vi "Camera.v2.vi"() -> ()   [LabVIEW 2015]
uses:
  CameraState.ctl
  Camera Properties.ctl
  <vilib>/vision/NI_Vision_Development_Module.lvlib
  CameraControlTypeDef.ctl
  Stack Track.ctl
  Stack_State.ctl
  ModeEnum.ctl
  <vilib>/DAQmx/create/channels.llb/DAQmx Create Channel (AO-Voltage-Basic).vi
  <vilib>/DAQmx/configure/timing.llb/DAQmx Timing (Sample Clock).vi
  WaveformModes.ctl
  <vilib>/DAQmx/write.llb/DAQmx Write (Digital 1D Wfm NChan NSamp).vi
  <vilib>/DAQmx/write.llb/DAQmx Write (Analog 1D Wfm NChan NSamp).vi
  Microscope Settings.ctl
panel:
  in  "Tab Control":enum32{"Camera Settings", "Recording"}(tab)
  in  "Scan":bool
  in  "Scan Continuously":bool
  in  "Camera Mode":T1(ring)
  in  "Slit Width /percent":dbl=100.0
  out "error IO":errorcluster
  in  "V Height":dbl=2048.0 min=4.0 max=2048.0 step=4.0
  in  "V Offset":dbl min=0.0 max=0.0 step=4.0
  in  "H Offset":dbl min=0.0 max=0.0 step=4.0
  in  "H Width":dbl min=4.0 max=2048.0 step=4.0
  in  "Exposure /ms":dbl=40.0 min=0.0010036691729323308 max=10.000004210526315 step=1e-08
  in  "Trigger Source":dbl(ring)=2.0 items=["Internal"=1.0, "External"=2.0]
  in  "Readout Direction":dbl(ring)=2.0 items=["Forward"=1.0, "Backward"=2.0]
  in  "Scanning Mode":dbl(ring)=12.0 items=["Full Frame"=1.0, "Slit Scanning"=12.0]
  in  "Advanced DCAM Controls":i32(listbox) caption="Multicolumn Listbox"
  in  "Mode":T2
  in  "FOV /um":dbl(slide) scale=-10.0..10.0
  in  "Mode":T3
  in  "Properties":T4=4211904 items=["SENSOR MODE"=4212128, "CCD MODE"=4212384, "READOUT MODE"=4211872, "ACTIVE VIEW INDEX"=4343136, "BITS PER CHANNEL"=4342976, "IMAGE PIXEL TYPE"=4343296, "BINNING"=4215968, "EXPOSURE TIME"=2049184, "CONTRAST GAIN"=3163312, "CONTRAST OFFSET"=3163328, "LIGHT MODE"=2114720, "SENSITIVITY"=2114992, "PHOTON IMAGING MODE"=2115200, "HIGH DYNAMIC RANGE MODE"=3163360, "WHITE BALANCE"=3163568, "TEMPERATURE"=2115232, "TEMPERATURE TARGET"=2115264, "SENSOR COOLER FAN"=2115296, "LINEBUNDLE HEIGHT"=4212192, "MECHANICAL SHUTTER"=2115488, "BACK FOCUS POSITION"=8422304, "TRIGGER CONNECTOR"=1066432, "TRIGGER SOURCE"=1066144, "OUTPUT TRIGGER SOURCE"=1852576, "TRIGGER GLOBAL EXPOSURE"=2049680, "FIRST TRIGGER BEHAVIOR"=2049696, "CHANNEL SYNC"=1852352, "READOUT DIRECTION"=4211904, "PRE HSYNC COUNT"=1852704, "INTERNAL LINE SPEED"=4191408, "INTERNAL LINE INVERVAL"=4191424]
  out "Image":T5(plugin-control)
  out "Histogram":T6(graph)
  in  "stop":bool
  in  "Calibration":bool
  in  "MultiD Scan":bool
  in  "Stage Controller":bool
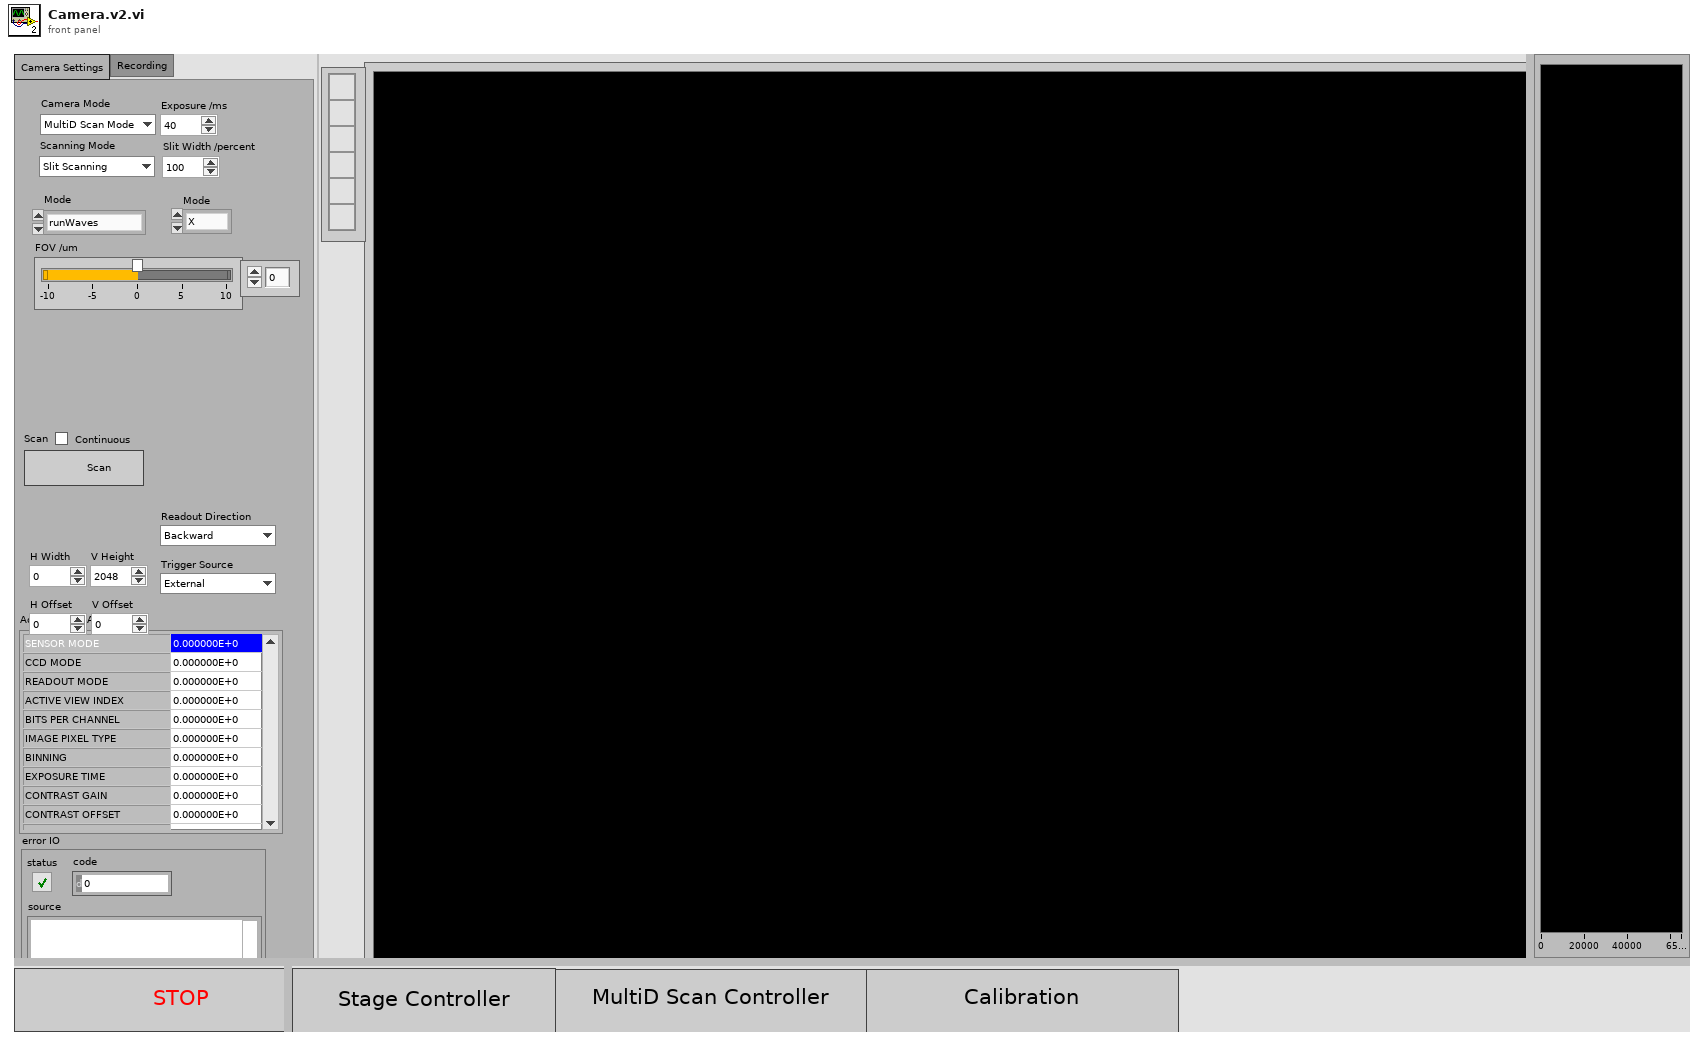
[diagram p1: front panel]
types:
  T1 = enum16{"MultiD Scan Mode", "2D Scan Mode", "Calibration Mode"}
  T2 = typedef "ModeEnum.ctl" = enum16{"runWaves", "generateWaves", "Idle", "stop"}
  T3 = typedef "WaveformModes.ctl" = enum16{"X", "XY", "XYZ", "XYZT", "XYZC"}
  T4 = typedef "Camera Properties.ctl" = u32
  T5 = typedef "IMAQ Image.ctl" = refnum<image>
  T6 = cluster{"Starting Value":sgl, "Incremental Value":sgl, "Histogram":u32[]}
  T7 = typedef "Microscope Settings.ctl" = cluster{"Mode":enum16{"X", "XY", "XYZ", "XYZT", "XYZC"}, "Piezo Position /um":dbl, "Exposure/ms":dbl, "Samples/millisecond":dbl, "Relax/ms":dbl}
  T8 = typedef "CameraControlTypeDef.ctl" = enum16{"IntervalLineInt", "Ram Record", "HardDisk Record", "Disengage Update", "Update", "Idle", "ROI", "Binning", "Scan Mode", "Trigger Mode", "Readout Mode", "Readout Direction", "Preview", "ROIWindow", "Trigger Source"}
  T9 = cluster{"height":u32, "width":u32, "datatype":u32}
  T10 = typedef "Stack_State.ctl" = cluster{"State":T11, "Stack Number":i32, "Image":u16[][], "Stacks":i32}
  T11 = typedef "Stack Track.ctl" = enum16{"Idle", "Display", "Start Sequence", "Read Disk", "STOP", "Collecting", "End"}
  T12 = typedef "CameraState.ctl" = enum16{"init", "active", "deinit"}
  T13 = typedef "Image Type" = u32
  T14 = cluster{"Value":i32, "Minimum":i32, "Maximum":i32, "Increment":i32}
  T15 = cluster{"Minimum":i32, "Maximum":i32, "Increment":i32}
  T16 = cluster{"Enum":T8, dbl, "timeout in ms (-1)":u32}
  T17 = cluster{"State":T11, "Timeout":i32, "Data 16":u16[][], "Timeout":i32}
  T18 = cluster{"Enum":T8, "Trigger Source":dbl, "timeout in ms (-1)":i32}
  T19 = cluster{"Enum":T8, "Exposure /ms":dbl, "Parameter":u32}
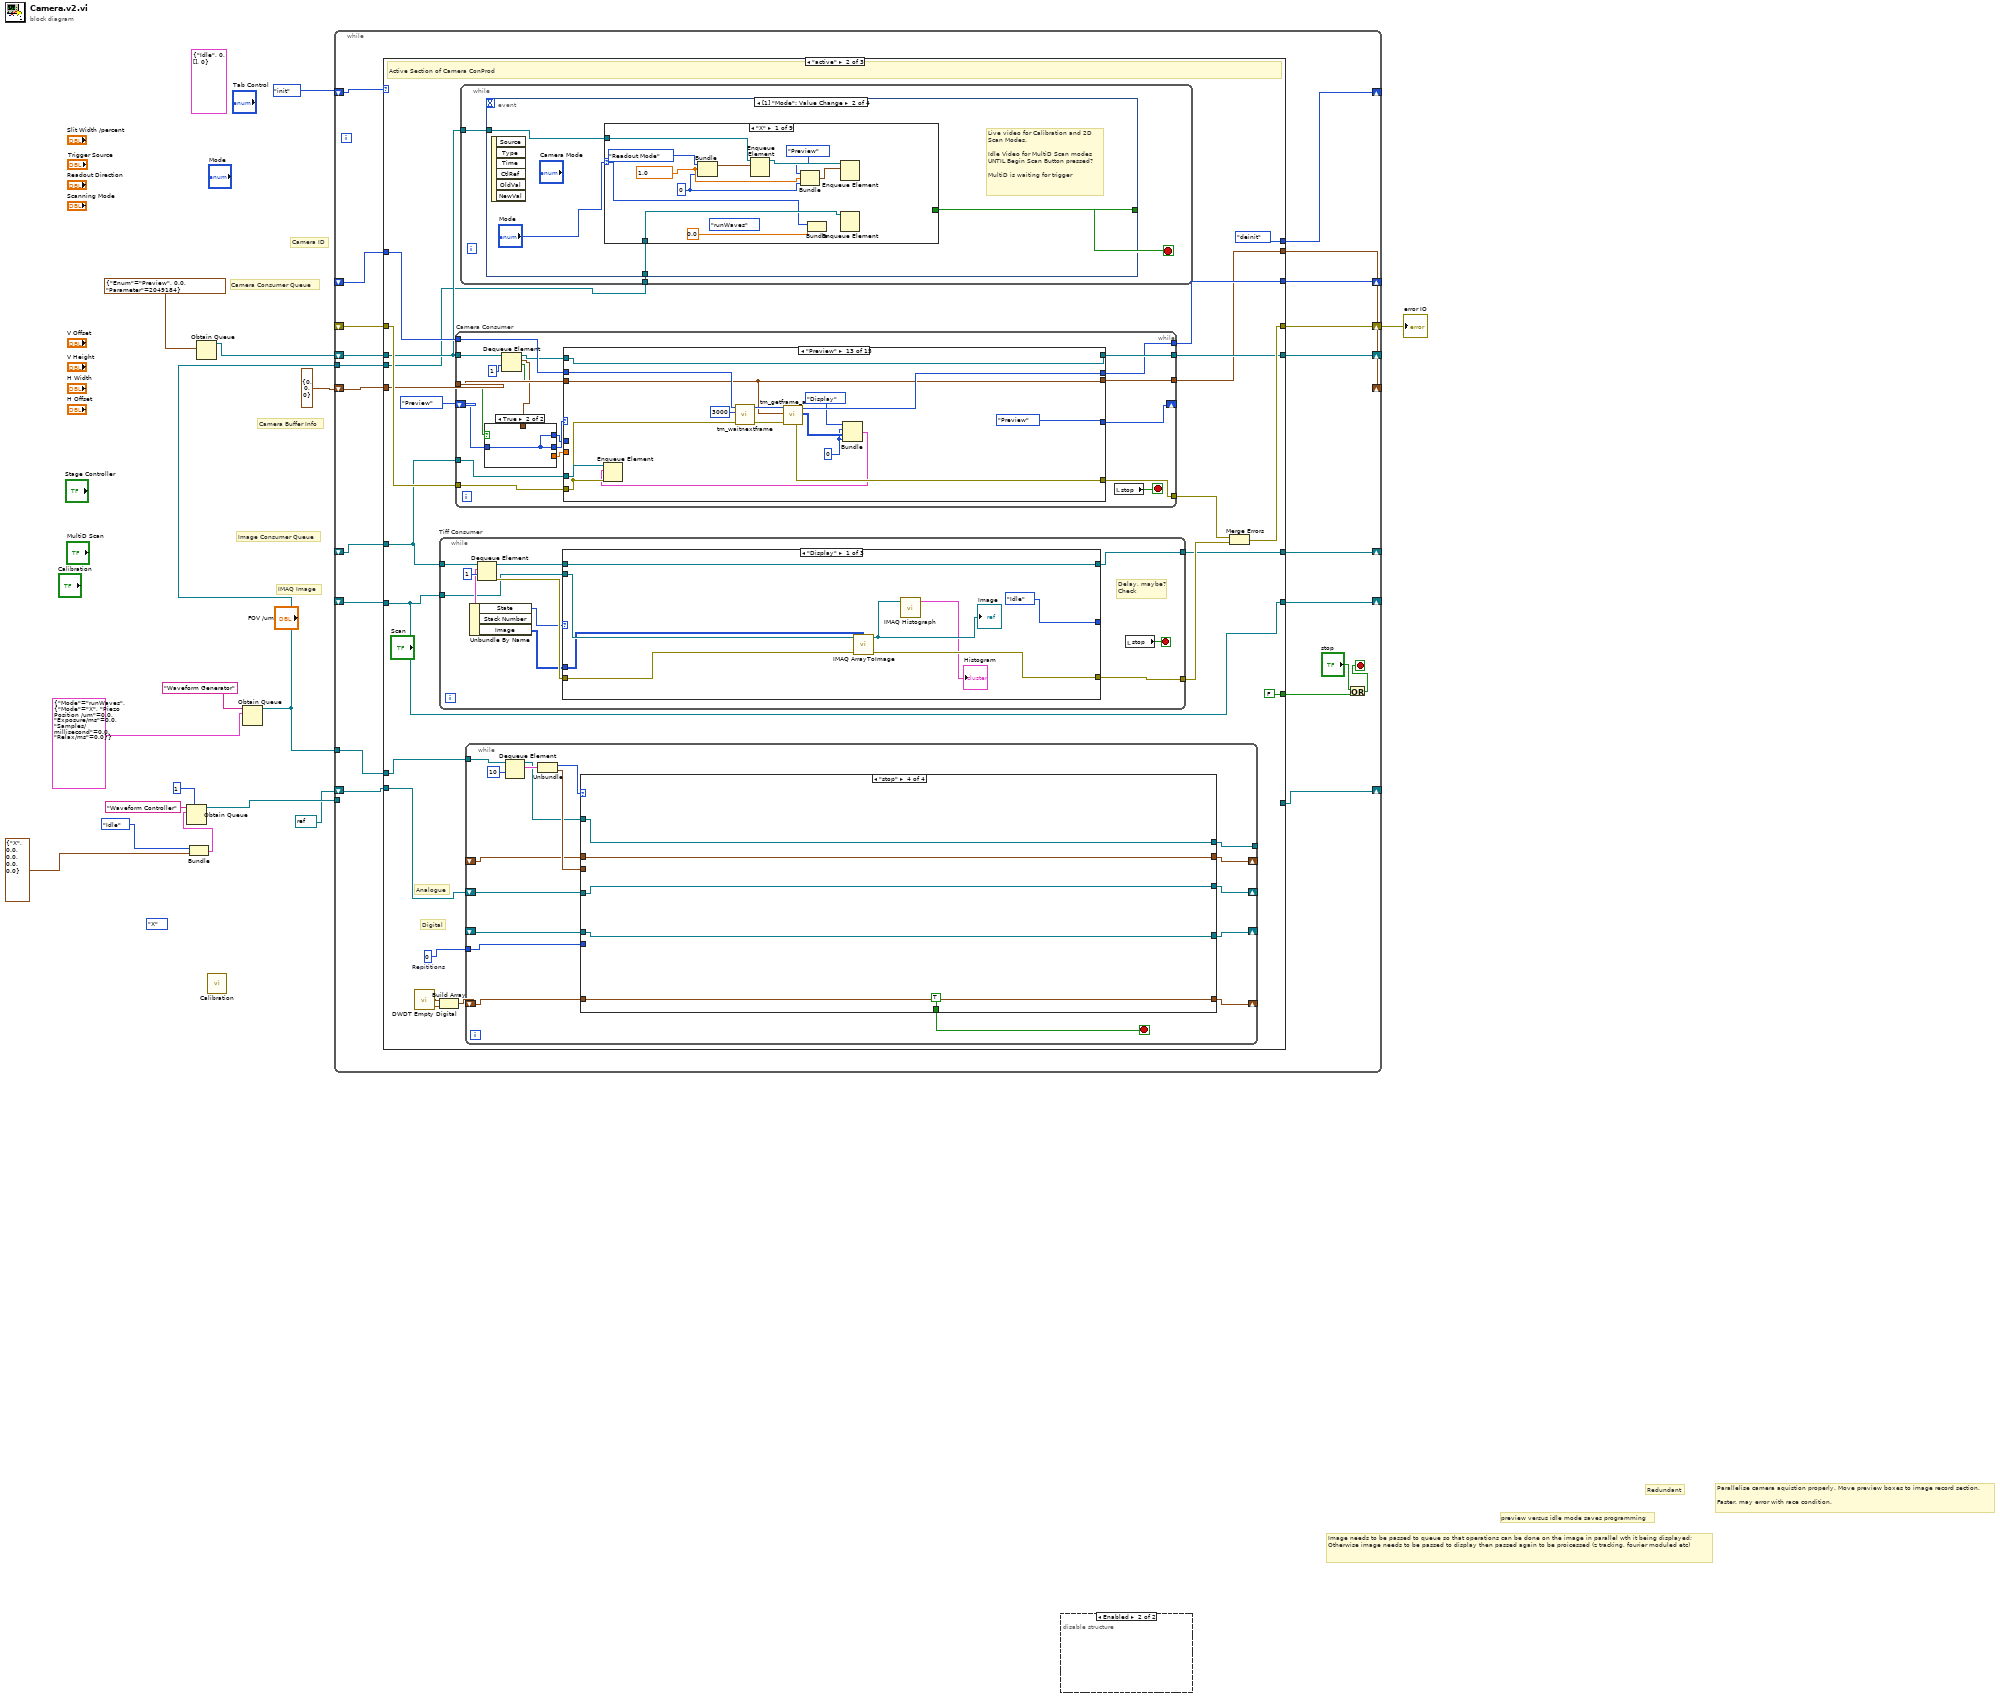
[diagram p0: block diagram]
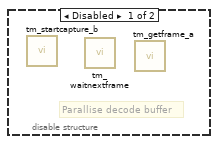
[diagram p2: hidden frame]
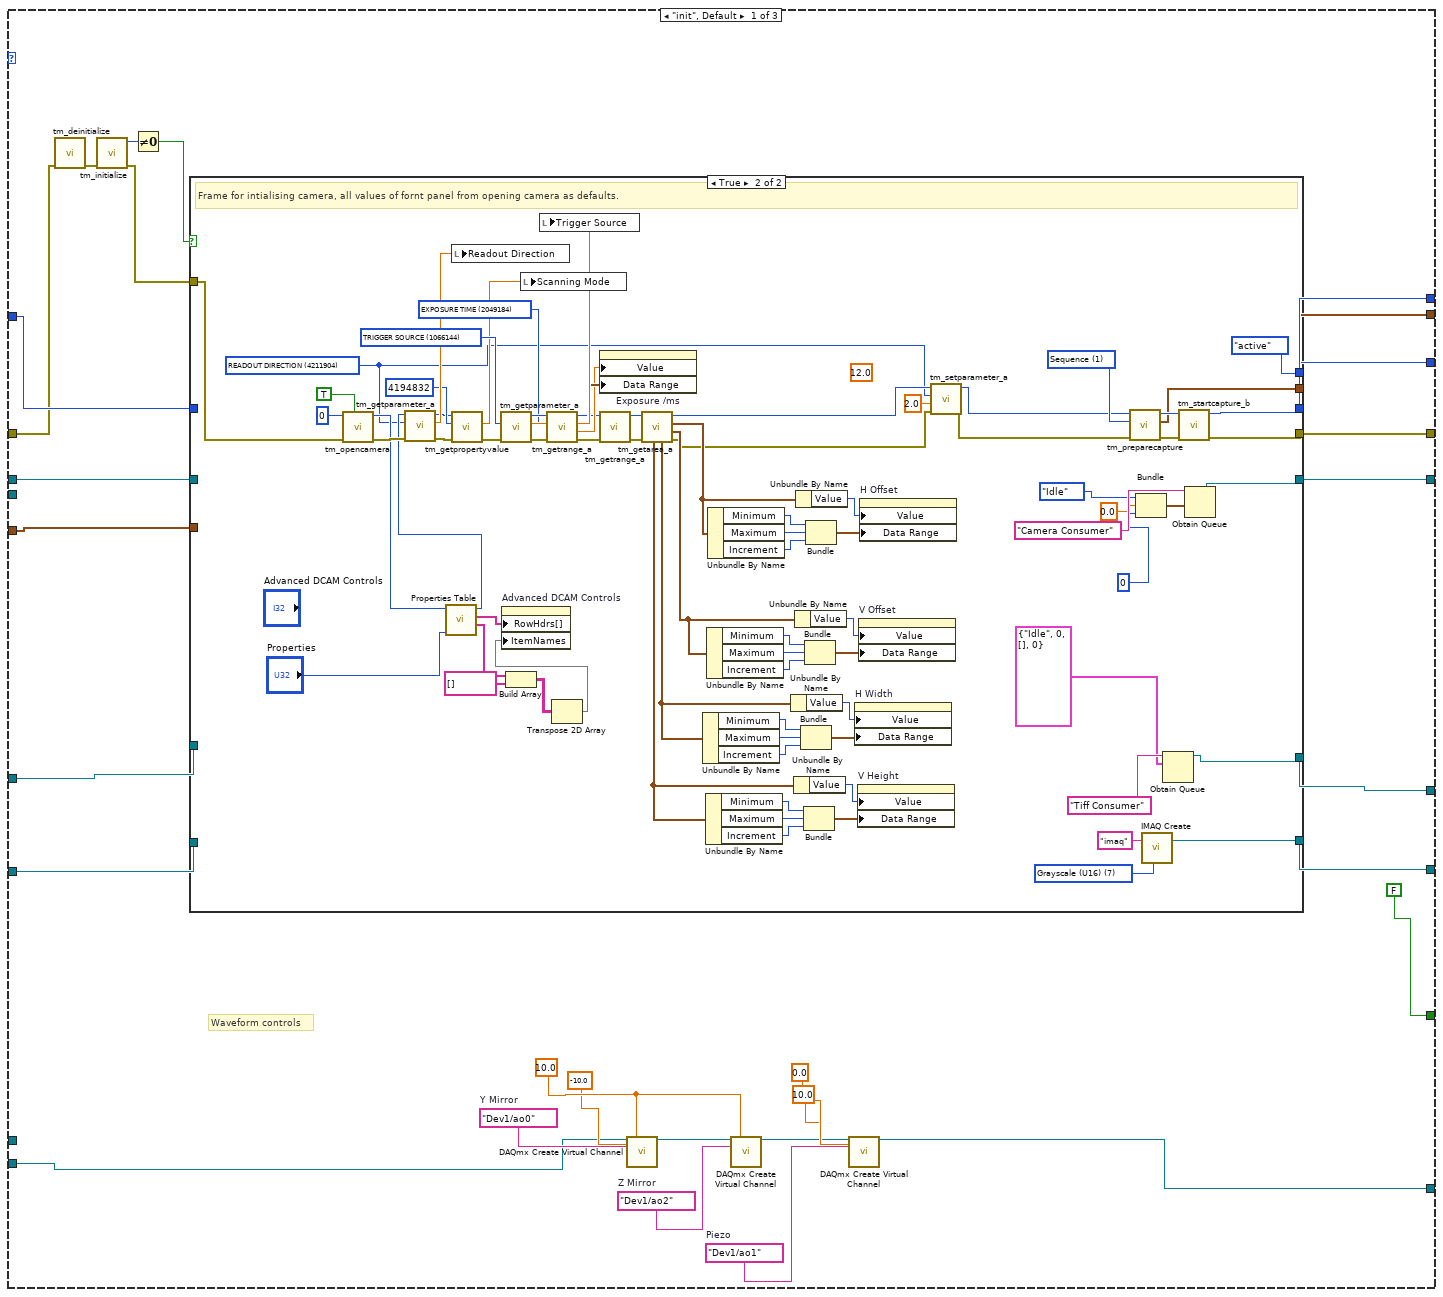
[diagram p3: hidden frame]
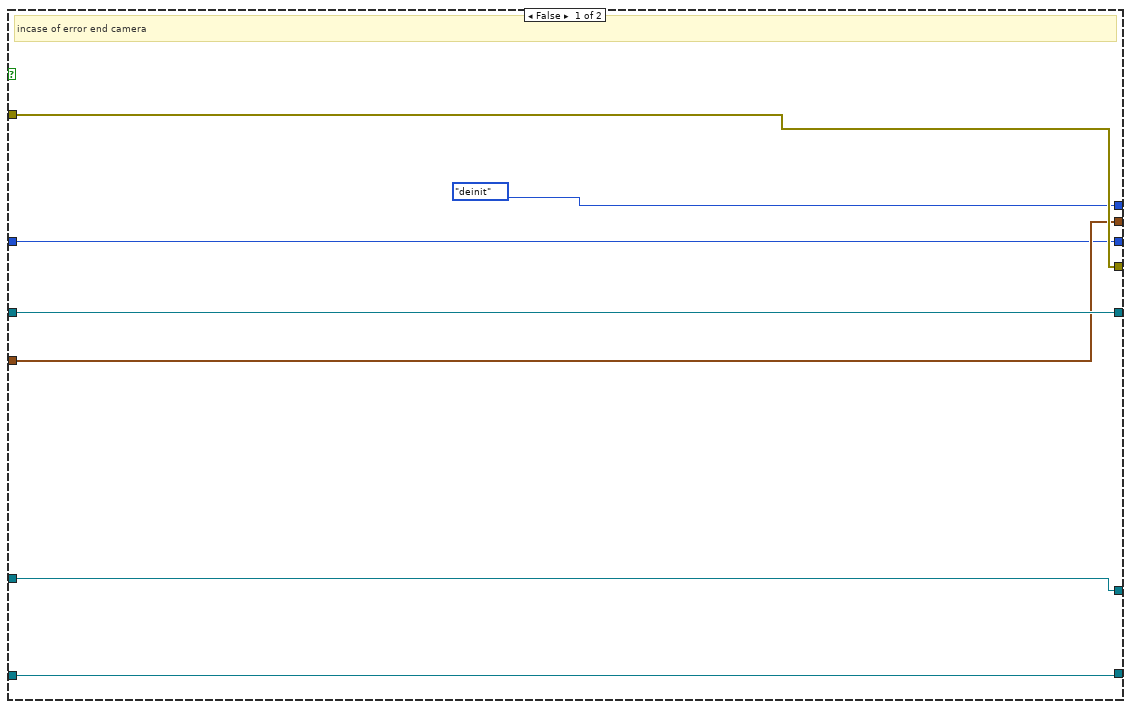
[diagram p4: hidden frame]
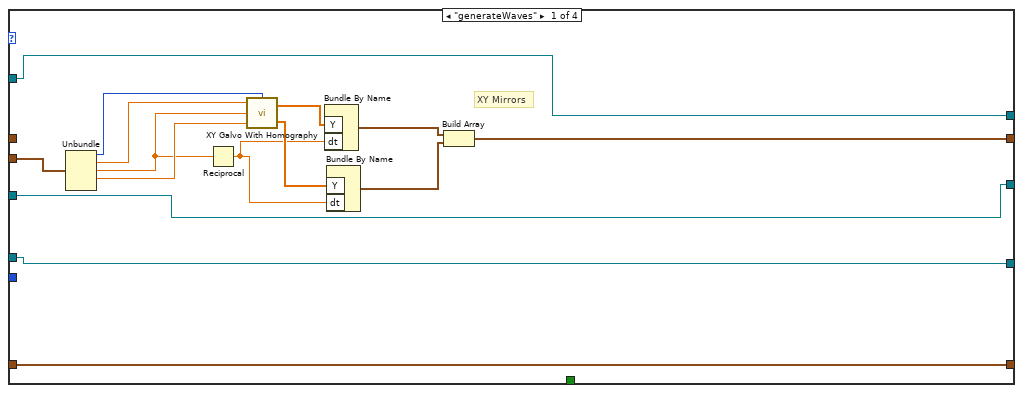
[diagram p5: hidden frame]
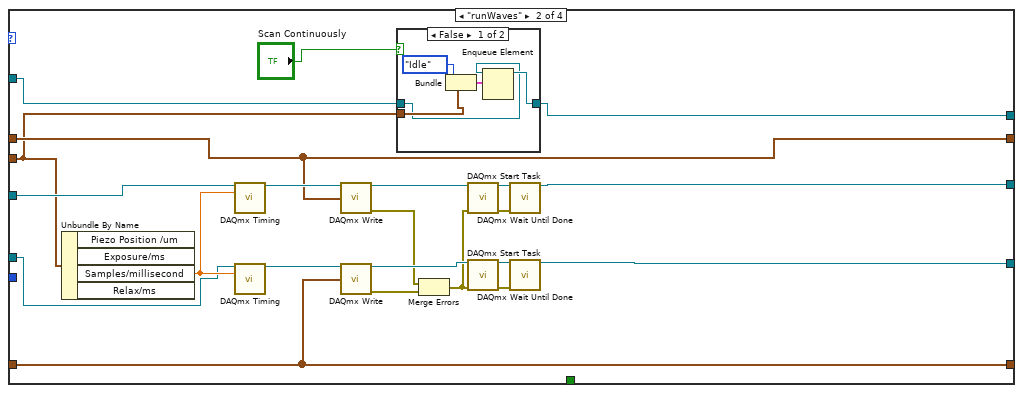
[diagram p6: hidden frame]
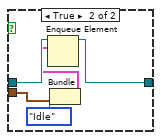
[diagram p7: hidden frame]
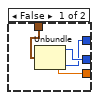
[diagram p11: hidden frame]
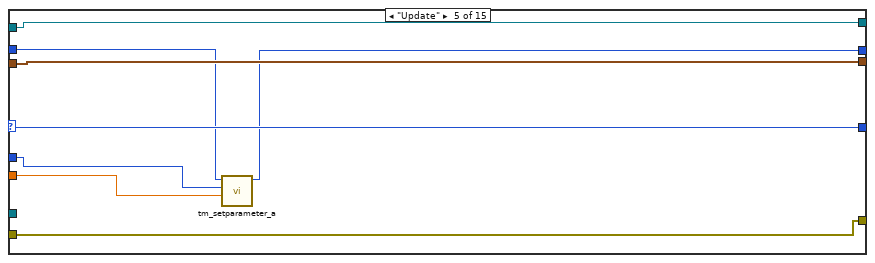
[diagram p16: hidden frame]
diagram:
  (unwired) WaveformModes."X"
  (unwired) T10 {"State"=enum."Idle", "Stack Number"=0, "Image"=[], "Stacks"=0} ("input cluster")
  # "IMAQ Image"
  # "Camera Buffer Info"
  # "Image needs to be passed to queue so that operations can be done on the image in parallel wth it being displayed;\nOtherwise image needs to be passed to display then passed again to be proicessed (z tracking, fourier moduled etc)"
  # "preview versus idle mode saves programming"
  # "Parallelise camera aquistion properly. Move preview boxes to image record section.\n\nFaster. may error with race condition."
  # "Redundant"
  # "Image Consumer Queue"
  # "Camera Consumer Queue"
  # "Camera ID"
  n1 = Bundle("Mode"=ModeEnum."Idle", T7 {"Mode"=enum."X", "Piezo Position /um"=0.0, "Exposure/ms"=0.0, "Samples/millisecond"=0.0, "Relax/ms"=0.0}) -> (w6:cluster{"Mode":T2, T7})  [unwired: 1 in]
  n2 = Obtain Queue(max queue size (-1, unlimited)=1, name (unnamed)="Waveform Controller", element data type=w6) -> (queue out=w3:refnum<queue>)  [unwired: 2 in, 2 out]
  n3 = Obtain Queue(element data type=cluster{"Enum":T8, dbl, "Parameter":u32} {"Enum"=enum."Preview", 0.0, "Parameter"=2049184}) -> (queue out=w10:refnum<queue>)  [unwired: 4 in, 2 out]
  n4 = call "Calibration.vi"() -> ()  [unwired: 1 in, 1 out]
  n5 = Obtain Queue(name (unnamed)="Waveform Generator", element data type=cluster{"Mode":T2, T7} {"Mode"=enum."runWaves", {"Mode"=enum."X", "Piezo Position /um"=0.0, "Exposure/ms"=0.0, "Samples/millisecond"=0.0, "Relax/ms"=0.0}}) -> (queue out=w9:refnum<queue>)  [unwired: 3 in, 2 out]
  n6 = while {
    shift-right: [w36] -> _
    shift-left: CameraState."init" -> [w35]
    shift-right: [w34] -> _
    shift-left: _ -> [w33]
    shift-right: [w32] -> w14
    shift-left: _ -> [w31]
    shift-right: [w29] -> _
    shift-left: _ -> [w28]
    shift-right: [w30] -> _
    shift-left: w10 -> [w27]
    shift-right: [w23] -> _
    shift-left: T9 {"height"=0, "width"=0, "datatype"=0} ("Buffer Info") -> [w22]
    shift-right: [w21] -> _
    shift-left: _ -> [w20]
    tunnel: w9 -> [w19]
    tunnel: w9 -> [w18]
    tunnel: w3 -> [_]
    shift-right: [w17] -> _
    shift-left: refnum<k21> refnum ("Mirror Z 2") -> [w16]
    stop <- w25 stop-if-true
    n7 = case shown="\"active\"" w35 {
      tunnel: [w61 CameraState."deinit" CameraState."init"] -> w36
      tunnel: [w60 w171 w445] -> w34
      tunnel: w33 -> [w38 w172 w445]
      tunnel: [w59 w170 w448] -> w32
      tunnel: w31 -> [w37 w164 w449]
      tunnel: [w58 w167 w442] -> w30
      tunnel: [w57 w166 w443] -> w29
      tunnel: w28 -> [w55 w159 w443]
      tunnel: w27 -> [w56 w157 w442]
      tunnel: [FALSE ("stop") FALSE ("stop") TRUE ("stop")] -> w24
      tunnel: [w53 w162 w440] -> w23
      tunnel: w22 -> [w52 w161 w440]
      tunnel: w20 -> [w50 w158 w439]
      tunnel: [w51 w158 w439] -> w21
      tunnel: w19 -> [_ w151 _]
      tunnel: w18 -> [_ w156 _]
      tunnel: [w42 _ w437] -> w17
      tunnel: w16 -> [w39 w152 w437]
      frame "init", Default {
        w45 = tag "Dev1/ao1"  # Piezo
        w46 = tag "Dev1/ao2"  # Z Mirror
        w47 = tag "Dev1/ao0"  # Y Mirror
        w49 = 10.0 ("maximum value")
        # "Waveform controls"
        n8 = call "tm_deinitialize.vi"("error in (no error)"=w37) -> ("error out"=w65:errorcluster)  [unwired: 10 in]
        n9 = call "tm_initialize.vi"("error in (no error)"=w65) -> ("error out"=w62:errorcluster, "Number Of Cameras"=w64:u32)  [unwired: 7 in, 2 out]
        n10 = Not Equal To 0?(x=w64) -> (x != 0?=w63:bool)
        n11 = case shown="True" w63 {
          tunnel: w62 -> [w72 w144]
          tunnel: [CameraState."deinit" CameraState."active"] -> w61
          tunnel: [w72 w127] -> w59
          tunnel: [w67 w125] -> w60
          tunnel: [w70 w99] -> w58
          tunnel: [w69 w97] -> w57
          tunnel: w56 -> [w70 _]
          tunnel: w55 -> [w69 _]
          tunnel: [w68 w87] -> w53
          tunnel: w52 -> [w68 _]
          tunnel: w38 -> [w67 _]
          tunnel: [w66 w84] -> w51
          tunnel: w50 -> [w66 _]
          frame False {
            # "incase of error end camera"
          }
          frame True {
            (unwired) 12.0 ("Value in")
            w86 = T13 7 items=["Grayscale (U8)", "Grayscale (I16)", "Grayscale (SGL)", "Complex (CSG)", "RGB (U32)", "HSL (U32)", "RGB (U64)", "Grayscale (U16)"] ("Image Type")
            w129 = 1 items=["Snap", "Sequence"] ("Capture mode")
            w141 = u32 2049184 items=["SENSOR MODE"=4212128, "CCD MODE"=4212384, "READOUT MODE"=4211872, "ACTIVE VIEW INDEX"=4343136, "BITS PER CHANNEL"=4342976, "IMAGE PIXEL TYPE"=4343296, "BINNING"=4215968, "EXPOSURE TIME"=2049184, "CONTRAST GAIN"=3163312, "CONTRAST OFFSET"=3163328, "LIGHT MODE"=2114720, "SENSITIVITY"=2114992, "PHOTON IMAGING MODE"=2115200, "HIGH DYNAMIC RANGE MODE"=3163360, "WHITE BALANCE"=3163568, "TEMPERATURE"=2115232, "TEMPERATURE TARGET"=2115264, "SENSOR COOLER FAN"=2115296, "LINEBUNDLE HEIGHT"=4212192, "MECHANICAL SHUTTER"=2115488, "BACK FOCUS POSITION"=8422304, "TRIGGER CONNECTOR"=1066432, "TRIGGER SOURCE"=1066144, "OUTPUT TRIGGER SOURCE"=1852576, "TRIGGER GLOBAL EXPOSURE"=2049680, "FIRST TRIGGER BEHAVIOR"=2049696, "CHANNEL SYNC"=1852352, "READOUT DIRECTION"=4211904, "PRE HSYNC COUNT"=1852704, "INTERNAL LINE SPEED"=4191408, "INTERNAL LINE INVERVAL"=4191424] ("Parameter")
            w79 = T4 4211904 items=["SENSOR MODE"=4212128, "CCD MODE"=4212384, "READOUT MODE"=4211872, "ACTIVE VIEW INDEX"=4343136, "BITS PER CHANNEL"=4342976, "IMAGE PIXEL TYPE"=4343296, "BINNING"=4215968, "EXPOSURE TIME"=2049184, "CONTRAST GAIN"=3163312, "CONTRAST OFFSET"=3163328, "LIGHT MODE"=2114720, "SENSITIVITY"=2114992, "PHOTON IMAGING MODE"=2115200, "HIGH DYNAMIC RANGE MODE"=3163360, "WHITE BALANCE"=3163568, "TEMPERATURE"=2115232, "TEMPERATURE TARGET"=2115264, "SENSOR COOLER FAN"=2115296, "LINEBUNDLE HEIGHT"=4212192, "MECHANICAL SHUTTER"=2115488, "BACK FOCUS POSITION"=8422304, "TRIGGER CONNECTOR"=1066432, "TRIGGER SOURCE"=1066144, "OUTPUT TRIGGER SOURCE"=1852576, "TRIGGER GLOBAL EXPOSURE"=2049680, "FIRST TRIGGER BEHAVIOR"=2049696, "CHANNEL SYNC"=1852352, "READOUT DIRECTION"=4211904, "PRE HSYNC COUNT"=1852704, "INTERNAL LINE SPEED"=4191408, "INTERNAL LINE INVERVAL"=4191424] ("Parameter")
            w147 = u32 1066144 items=["SENSOR MODE"=4212128, "CCD MODE"=4212384, "READOUT MODE"=4211872, "ACTIVE VIEW INDEX"=4343136, "BITS PER CHANNEL"=4342976, "IMAGE PIXEL TYPE"=4343296, "BINNING"=4215968, "EXPOSURE TIME"=2049184, "CONTRAST GAIN"=3163312, "CONTRAST OFFSET"=3163328, "LIGHT MODE"=2114720, "SENSITIVITY"=2114992, "PHOTON IMAGING MODE"=2115200, "HIGH DYNAMIC RANGE MODE"=3163360, "WHITE BALANCE"=3163568, "TEMPERATURE"=2115232, "TEMPERATURE TARGET"=2115264, "SENSOR COOLER FAN"=2115296, "LINEBUNDLE HEIGHT"=4212192, "MECHANICAL SHUTTER"=2115488, "BACK FOCUS POSITION"=8422304, "TRIGGER CONNECTOR"=1066432, "TRIGGER SOURCE"=1066144, "OUTPUT TRIGGER SOURCE"=1852576, "TRIGGER GLOBAL EXPOSURE"=2049680, "FIRST TRIGGER BEHAVIOR"=2049696, "CHANNEL SYNC"=1852352, "READOUT DIRECTION"=4211904, "PRE HSYNC COUNT"=1852704, "INTERNAL LINE SPEED"=4191408, "INTERNAL LINE INVERVAL"=4191424] ("Parameter")
            # "Frame for intialising camera, all values of fornt panel from opening camera as defaults."
            n12 = call "tm_opencamera.vi"("Force Open"=TRUE, "error in (no error)"=w144, "Camera Index"=u32 0) -> ("error out"=w148:errorcluster, "Handle out"=w95:u32)  [unwired: 6 in, 1 out]
            n13 = call "Properties Table.vi"("Properties"="Properties", "Handle In"=w95) -> ("Value Stirngs Out"=w92:string[], "Row Headers"=w93:string[], "Handle Out"=w94:u32)  [unwired: 3 in, 1 out]
            n14 = call "tm_getparameter_a.vi"("error in (no error)"=w148, "Parameter"=w79, "Handle in"=w94) -> ("error out"=w130:errorcluster, "Value out"=w145:dbl, "Handle out"=w133:u32)  [unwired: 6 in]
            n15 = local write "Readout Direction"(w145) -> ()
            n16 = call "tm_getpropertyvalue.vi"("error in (no error)"=w130, "Property ID"=u32 4194832, "Handle in"=w133) -> ("error out"=w131:errorcluster, "Value in"=w132:sgl)  [unwired: 6 in, 1 out]
            n17 = call "tm_getparameter_a.vi"("error in (no error)"=w131, "Parameter"=w147) -> ("error out"=w142:errorcluster, "Value out"=w146:dbl, "Handle out"=w143:u32)  [unwired: 7 in]
            n18 = Build Array(w92, string[] [] ("element")) -> (w90:string[][])
            n19 = local write "Scanning Mode"(w132) -> ()
            n20 = local write "Trigger Source"(w146) -> ()
            n21 = call "tm_getrange_a.vi"("error in (no error)"=w142, "Parameter"=w141, "Handle in"=w143) -> ("error out"=w137:errorcluster, "default"=w139:dbl, "Range"=w140:cluster{"min":dbl, "max":dbl, "step":dbl}, "Handle out"=w138:u32)  [unwired: 2 in, 3 out]
            n22 = Transpose 2D Array(2D array=w90) -> (transposed array=w89:string[][])
            n23 = property on="Advanced DCAM Controls" class="MCListbox (strict)"("RowHdrs[]"=w93, "ItemNames"=w89) -> ()  [unwired: 2 in, 2 out]
            n24 = property on="Exposure /ms" class="DigNum (strict)"("Value"=w139, "Data Range"=w140) -> ()  [unwired: 2 in, 2 out]
            n25 = call "tm_getrange_a.vi"("error in (no error)"=w137, "Handle in"=w138) -> ("error out"=w136:errorcluster, "Handle out"=w135:u32)  [unwired: 3 in, 5 out]
            n26 = call "tm_getarea_a.vi"("error in (no error)"=w136, "Handle in"=w135) -> ("error out"=w81:errorcluster, "V Offset"=w101:T14, "H Offset"=w124:T14, "Handle out"=w83:u32, "H Width"=w102:T14, "V Width"=w103:T14)  [unwired: 4 in]
            n27 = Unbundle By Name(w102) -> ("Minimum"=w113:i32, "Maximum"=w112:i32, "Increment"=w111:i32)
            n28 = Unbundle By Name(w103) -> ("Minimum"=w104:i32, "Maximum"=w105:i32, "Increment"=w106:i32)
            n29 = Unbundle By Name(w101) -> ("Minimum"=w114:i32, "Maximum"=w115:i32, "Increment"=w116:i32)
            n30 = Unbundle By Name(w124) -> ("Minimum"=w123:i32, "Maximum"=w122:i32, "Increment"=w121:i32)
            n31 = Unbundle By Name(w102) -> ("Value"=w109:i32)
            n32 = Unbundle By Name(w103) -> ("Value"=w108:i32)
            n33 = Unbundle By Name(w101) -> ("Value"=w118:i32)
            n34 = Unbundle By Name(w124) -> ("Value"=w119:i32)
            n35 = Bundle("Minimum"=w113, "Maximum"=w112, "Increment"=w111) -> (w110:T15)  [unwired: 1 in]
            n36 = Bundle("Minimum"=w104, "Maximum"=w105, "Increment"=w106) -> (w107:T15)  [unwired: 1 in]
            n37 = Bundle("Minimum"=w114, "Maximum"=w115, "Increment"=w116) -> (w117:T15)  [unwired: 1 in]
            n38 = Bundle("Minimum"=w123, "Maximum"=w122, "Increment"=w121) -> (w120:T15)  [unwired: 1 in]
            n39 = property on="H Width" class="DigNum (strict)"("Value"=w109, "Data Range"=w110) -> ()  [unwired: 2 in, 2 out]
            n40 = property on="V Height" class="DigNum (strict)"("Value"=w108, "Data Range"=w107) -> ()  [unwired: 2 in, 2 out]
            n41 = property on="V Offset" class="DigNum (strict)"("Value"=w118, "Data Range"=w117) -> ()  [unwired: 2 in, 2 out]
            n42 = property on="H Offset" class="DigNum (strict)"("Value"=w119, "Data Range"=w120) -> ()  [unwired: 2 in, 2 out]
            n43 = call "tm_setparameter_a.vi"("error in (no error)"=w81, "Value in"=2.0, "Parameter"=w79, "Handle in"=w83) -> ("error out"=w80:errorcluster, "Handle out"=w82:u32)  [unwired: 6 in]
            n44 = call "tm_preparecapture.vi"("error in (no error)"=w80, "Capture mode"=w129, "Handle in"=w82) -> ("error out"=w128:errorcluster, "Buffer Info"=w87:T9, "Handle out"=w126:u32)  [unwired: 5 in, 1 out]
            n45 = Bundle("Enum"=CameraControlTypeDef."Idle", 0.0, "timeout in ms (-1)"=u32 0) -> (w75:T16)  [unwired: 1 in]
            n46 = call "IMAQ Create"("Image Name"="imaq", "Image Type"=w86) -> ("New Image"=w84:T5)  [unwired: 3 in, 1 out]
            n47 = Obtain Queue(name (unnamed)="Tiff Consumer", element data type=T10 {"State"=enum."Idle", "Stack Number"=0, "Image"=[], "Stacks"=0} ("input cluster")) -> (queue out=w97:refnum<queue>)  [unwired: 3 in, 2 out]
            n48 = call "tm_startcapture_b.vi"("error in (no error)"=w128, "Handle in"=w126) -> ("error out"=w127:errorcluster, "Handle out"=w125:u32)  [unwired: 8 in]
            n49 = Obtain Queue(name (unnamed)="Camera Consumer", element data type=w75) -> (queue out=w99:refnum<queue>)  [unwired: 3 in, 2 out]
          }
        }
        n50 = call-poly <vilib>:"DAQmx Create Virtual Channel.vi"("task in"=w39, "maximum value"=w49, "minimum value"=-10.0, "physical channels"=w47) -> ("task out"=w41:refnum<k21>)  [unwired: 10 in, 1 out]
        n51 = call-poly <vilib>:"DAQmx Create Virtual Channel.vi"("task in"=w41, "maximum value"=w49, "physical channels"=w46) -> ("task out"=w40:refnum<k21>)  [unwired: 11 in, 1 out]
        n52 = call-poly <vilib>:"DAQmx Create Virtual Channel.vi"("task in"=w40, "maximum value"=10.0 ("minimum value"), "minimum value"=0.0 ("maximum value"), "physical channels"=w45) -> ("task out"=w42:refnum<k21>)  [unwired: 10 in, 1 out]
      }
      frame "active" {
        w155 = 0  # Repititions
        # "Digital"
        # "Analogue"
        # "Active Section of Camera ConProd"
        n53 = call <vilib>:"DWDT Empty Digital.vi"() -> ("digital waveform out"=w153:digitalwaveform)  [unwired: 5 in]
        n54 = while "Tiff Consumer" {
          tunnel: [w251] -> w169
          tunnel: [w254] -> w166
          tunnel: w159 -> [w256]
          tunnel: w158 -> [w248]
          stop <- w258 stop-if-true
          # "Delay, maybe?\nCheck"
          n55 = Dequeue Element(queue=w256, timeout in ms (-1)=1) -> (queue out=w253:refnum<queue>, element=w255:T10, error out=w252:errorcluster)  [unwired: 1 in, 1 out]
          n56 = Unbundle By Name(w255) -> ("State"=w249:T11, "Image"=w250:u16[][])  [unwired: 1 out]
          n57 = case shown="\"Display\"" w249 {
            selector: w249 -> [_ w269 w270]
            tunnel: [w266 w268 w271] -> w254
            tunnel: w253 -> [w266 w268 w271]
            tunnel: [Stack_Track."Idle" ("State") w269 w270] -> _
            tunnel: w250 -> [w261 _ _]
            tunnel: w248 -> [w265 _ _]
            tunnel: w252 -> [w264 w267 w272]
            tunnel: [w263 w267 w272] -> w251
            frame "Display" {
              n58 = call "IMAQ ArrayToImage"("Image Pixels (U16)"=w261, "error in (no error)"=w264, "Image"=w265) -> ("error out"=w263:errorcluster, "Image Out"=w260:T5)  [unwired: 7 in]
              "Image" <- w260
              n59 = call "IMAQ Histograph"("Image"=w260) -> ("Histogram Graph"=→"Histogram":T6)  [unwired: 7 in, 3 out]
            }
            frame "Idle", Default {
            }
            frame "Start Sequence" {
            }
          }
          n60 = local read "stop"() -> (w258:bool)
        }
        n61 = Build Array(w153, w153) -> (w154:digitalwaveform[])
        n62 = while "Camera Consumer" {
          tunnel: w164 -> [w289]
          tunnel: w172 -> [w286]
          tunnel: [w285] -> w171
          tunnel: [w288] -> w168
          tunnel: w157 -> [w281]
          tunnel: [w290] -> w167
          shift-right: [w287] -> _
          shift-left: CameraControlTypeDef."Preview" ("Enum") -> [w277]
          tunnel: [w284] -> w162
          tunnel: w161 -> [w283]
          tunnel: w159 -> [w276]
          stop <- w291 stop-if-true
          n63 = Dequeue Element(queue=w281, timeout in ms (-1)=1) -> (queue out=w280:refnum<queue>, element=w275:cluster{"Enum":T8, dbl, "Parameter":u32}, timed out?=w279:bool)  [unwired: 1 in, 1 out]
          n64 = case shown="True" w279 {
            tunnel: [w294 w296] -> w278
            tunnel: w277 -> [_ w296]
            tunnel: w275 -> [w295 _]
            tunnel: [w293 _] -> w274
            tunnel: [w292 w296] -> w273
            frame False {
              n65 = Unbundle(w295) -> ("Enum"=w294:T8, w293:dbl, "Parameter"=w292:u32)
            }
            frame True {
            }
          }
          n66 = case shown="\"Preview\"" w278 {
            selector: w278 -> [w300 w305 w310 w315 w323 w328 w333 w338 w343 w348 w353 w358 _ w377 _]
            tunnel: w280 -> [w299 w306 w311 w316 w324 w329 w334 w339 w344 w349 w354 w359 w374 w379 w384]
            tunnel: [w299 w306 w311 w316 w324 w329 w334 w339 w344 w349 w354 w359 w374 w379 w384] -> w290
            tunnel: w289 -> [w301 w304 w309 w314 w322 w327 w332 w337 w342 w347 w352 w357 w364 w376 w382]
            tunnel: [w301 w304 w309 w314 w322 w327 w332 w337 w342 w347 w352 w357 w368 w376 w382] -> w288
            tunnel: [w300 w305 w310 w315 w323 w328 w333 w338 w343 w348 w353 w358 CameraControlTypeDef."Preview" ("Enum") w377 CameraControlTypeDef."Preview" ("Enum")] -> w287
            tunnel: w286 -> [w298 w303 w308 w313 w320 w326 w331 w336 w341 w346 w351 w356 w372 w378 w383]
            tunnel: [w298 w303 w308 w313 w319 w326 w331 w336 w341 w346 w351 w356 w370 w378 w383] -> w285
            tunnel: [w297 w302 w307 w312 w321 w325 w330 w335 w340 w345 w350 w355 w366 w375 w381] -> w284
            tunnel: w283 -> [w297 w302 w307 w312 w321 w325 w330 w335 w340 w345 w350 w355 w366 w375 w381]
            tunnel: w276 -> [_ _ _ _ _ _ _ _ _ _ _ _ w365 _ _]
            tunnel: w274 -> [_ _ _ _ w317 _ _ _ _ _ _ _ _ _ _]
            tunnel: w273 -> [_ _ _ _ w318 _ _ _ _ _ _ _ _ _ _]
            frame "IntervalLineInt" {
            }
            frame "Ram Record" {
            }
            frame "HardDisk Record" {
            }
            frame "Disengage Update" {
            }
            frame "Update" {
              n67 = call "tm_setparameter_a.vi"("Value in"=w317, "Parameter"=w318, "Handle in"=w320) -> ("Handle out"=w319:u32)  [unwired: 7 in, 1 out]
            }
            frame "Idle", Default {
            }
            frame "ROI" {
            }
            frame "Binning" {
            }
            frame "Scan Mode" {
            }
            frame "Trigger Mode" {
            }
            frame "Readout Mode" {
            }
            frame "Readout Direction" {
            }
            frame "Preview" {
              w361 = 0 ("Timeout")
              n68 = call "tm_waitnextframe.vi"("error in (no error)"=w364, "Timeout"=3000, "Handle in"=w372) -> ("error out"=w369:errorcluster, "Handle out"=w371:u32)  [unwired: 5 in, 2 out]
              n69 = call "tm_getframe_a.vi"("error in (no error)"=w369, "Buffer Info"=w366, "Handle in"=w371) -> ("error out"=w368:errorcluster, "Data 16"=w362:u16[][], "Handle out"=w370:u32)  [unwired: 4 in, 2 out]
              n70 = Bundle("State"=Stack_Track."Display", "Timeout"=w361, "Data 16"=w362, "Timeout"=w361) -> (w360:T17)  [unwired: 1 in]
              n71 = Enqueue Element(queue=w365, element=w360, error in (no error)=w364) -> ()  [unwired: 1 in, 3 out]
            }
            frame "ROIWindow" {
            }
            frame "Trigger Source" {
              n72 = call "tm_unpreparecapture.vi"() -> ()  [unwired: 10 in, 2 out]
              n73 = call "tm_setparameter_a.vi"() -> ()  [unwired: 10 in, 2 out]
              n74 = call "tm_preparecapture.vi"() -> ()  [unwired: 8 in, 4 out]
            }
          }
          n75 = local read "stop"() -> (w291:bool)
        }
        n76 = while {
          tunnel: w157 -> [w386]
          tunnel: w156 -> [w385]
          stop <- w387 stop-if-true
          n77 = event shown="[1] \"Mode\": Value Change" {
            selector: _ -> [_ _ _ _]
            dyn-events: _ -> [_ _ _ _]
            timeout: _ -> [_ _ _ _]
            tunnel: [w388 w390 _ _] -> w387
            tunnel: w386 -> [_ w392 _ w435]
            tunnel: w385 -> [_ w391 _ w432]
            event "stop": Value Change {
              n78 = event-data() -> ()  [unwired: 1 in, 6 out]
              n79 = local read "stop"() -> (w388:bool)
            }
            event Value Change {
              # "Live video for Calibration and 2D\nScan Modes.\n\nIdle Video for MultiD Scan modes\nUNTIL Begin Scan Button pressed?\n\nMultiD is waiting for trigger"
              n80 = event-data() -> ()  [unwired: 1 in, 6 out]
              n81 = case shown="\"X\"" "Mode" {
                selector: "Mode" -> [w394 _ _ _ w417 _ _ _ _]
                tunnel: w392 -> [w402 w410 _ _ w425 _ _ _ _]
                tunnel: w391 -> [w395 _ w413 _ w416 _ _ _ _]
                tunnel: [_ _ _ _ _ TRUE FALSE _ _] -> w390
                frame "X" {
                  (unwired) ModeEnum."runWaves" ("Mode")
                  w396 = 0 ("timeout in ms (-1)")
                  w397 = 1.0 items=["Internal"=1.0, "External"=2.0] ("Trigger Source")
                  n82 = Bundle("Enum"=CameraControlTypeDef."Readout Mode", "Trigger Source"=w397, "timeout in ms (-1)"=w396) -> (w401:T18)  [unwired: 1 in]
                  n83 = Enqueue Element(queue=w402, element=w401) -> (queue out=w399:refnum<queue>)  [unwired: 2 in, 2 out]
                  n84 = Bundle("Enum"=CameraControlTypeDef."Preview", "Trigger Source"=w397, "timeout in ms (-1)"=w396) -> (w400:T18)  [unwired: 1 in]
                  n85 = Bundle("Mode"=w394, "Exposure /ms"=0.0) -> ()  [unwired: 1 in, 1 out]
                  n86 = Enqueue Element(queue=w399, element=w400) -> ()  [unwired: 2 in, 3 out]
                  n87 = Enqueue Element(queue=w395) -> ()  [unwired: 3 in, 3 out]
                }
                frame "XYZ" {
                  w404 = 0 ("timeout in ms (-1)")
                  w405 = 2.0 items=["Internal"=1.0, "External"=2.0] ("Trigger Source")
                  n88 = Bundle("Enum"=CameraControlTypeDef."Readout Mode", "Trigger Source"=w405, "timeout in ms (-1)"=w404) -> (w409:T18)  [unwired: 1 in]
                  n89 = Enqueue Element(queue=w410, element=w409) -> (queue out=w408:refnum<queue>)  [unwired: 2 in, 2 out]
                  n90 = Bundle("Enum"=CameraControlTypeDef."Idle", "Trigger Source"=w405, "timeout in ms (-1)"=w404) -> (w407:T18)  [unwired: 1 in]
                  n91 = Enqueue Element(queue=w408, element=w407) -> ()  [unwired: 2 in, 3 out]
                }
                frame "XYZT" {
                  w415 = ModeEnum."generateWaves"  # Mode
                  n92 = local read "Exposure /ms"() -> (w414:dbl)
                  n93 = Bundle("Mode"=w415, "Exposure /ms"=w414) -> (w412:cluster{"Mode":T2, "Exposure /ms":dbl})  [unwired: 1 in]
                  n94 = Enqueue Element(queue=w413, element=w412) -> ()  [unwired: 2 in, 3 out]
                }
                frame "XYZT" {
                }
                frame "XY" {
                  w419 = 0 ("timeout in ms (-1)")
                  w420 = 2.0 items=["Internal"=1.0, "External"=2.0] ("Trigger Source")
                  n95 = local read "Exposure /ms"() -> (w418:dbl)
                  n96 = Bundle("Enum"=CameraControlTypeDef."Readout Mode", "Trigger Source"=w420, "timeout in ms (-1)"=w419) -> (w424:T18)  [unwired: 1 in]
                  n97 = Enqueue Element(queue=w425, element=w424) -> (queue out=w421:refnum<queue>)  [unwired: 2 in, 2 out]
                  n98 = Bundle("Mode"=w417, "Exposure /ms"=w418) -> ()  [unwired: 1 in, 1 out]
                  n99 = Bundle("Enum"=CameraControlTypeDef."Preview", "Trigger Source"=w420, "timeout in ms (-1)"=w419) -> (w423:T18)  [unwired: 1 in]
                  n100 = Enqueue Element(queue=w416) -> ()  [unwired: 3 in, 3 out]
                  n101 = Enqueue Element(queue=w421, element=w423) -> ()  [unwired: 2 in, 3 out]
                }
                frame "XYZC" {
                }
                frame "XYZ" {
                }
                frame "XY" {
                }
                frame "X" {
                }
              }
            }
            event "Scan": Value Change {
              n102 = event-data() -> ()  [unwired: 1 in, 6 out]
            }
            event "Exposure /ms": Value Change {
              w431 = ModeEnum."generateWaves"  # Mode
              w433 = u32 2049184 items=["SENSOR MODE"=4212128, "CCD MODE"=4212384, "READOUT MODE"=4211872, "ACTIVE VIEW INDEX"=4343136, "BITS PER CHANNEL"=4342976, "IMAGE PIXEL TYPE"=4343296, "BINNING"=4215968, "EXPOSURE TIME"=2049184, "CONTRAST GAIN"=3163312, "CONTRAST OFFSET"=3163328, "LIGHT MODE"=2114720, "SENSITIVITY"=2114992, "PHOTON IMAGING MODE"=2115200, "HIGH DYNAMIC RANGE MODE"=3163360, "WHITE BALANCE"=3163568, "TEMPERATURE"=2115232, "TEMPERATURE TARGET"=2115264, "SENSOR COOLER FAN"=2115296, "LINEBUNDLE HEIGHT"=4212192, "MECHANICAL SHUTTER"=2115488, "BACK FOCUS POSITION"=8422304, "TRIGGER CONNECTOR"=1066432, "TRIGGER SOURCE"=1066144, "OUTPUT TRIGGER SOURCE"=1852576, "TRIGGER GLOBAL EXPOSURE"=2049680, "FIRST TRIGGER BEHAVIOR"=2049696, "CHANNEL SYNC"=1852352, "READOUT DIRECTION"=4211904, "PRE HSYNC COUNT"=1852704, "INTERNAL LINE SPEED"=4191408, "INTERNAL LINE INTERVAL"=4191424] ("Parameter")
              n103 = event-data() -> ()  [unwired: 1 in, 6 out]
              n104 = Bundle("Enum"=CameraControlTypeDef."Update", "Exposure /ms"="Exposure /ms", "Parameter"=w433) -> (w434:T19)  [unwired: 1 in]
              n105 = Enqueue Element(queue=w435, element=w434) -> ()  [unwired: 2 in, 3 out]
              n106 = Bundle("Mode"=w431, "Exposure /ms"="Exposure /ms") -> (w429:cluster{"Mode":T2, "Exposure /ms":dbl})  [unwired: 1 in]
              n107 = Enqueue Element(queue=w432, element=w429) -> ()  [unwired: 2 in, 3 out]
            }
          }
        }
        n108 = while {
          tunnel: w151 -> [w189]
          shift-right: [w184] -> _
          shift-left: _ -> [w183]
          tunnel: w155 -> [w182]
          tunnel: [w180] -> _
          shift-right: [w176] -> _
          shift-left: w152 -> [w175]
          shift-right: [w179] -> _
          shift-left: w154 -> [w178]
          shift-right: [w174] -> _
          shift-left: _ -> [w173]
          stop <- w188 stop-if-true
          n109 = Dequeue Element(queue=w189, timeout in ms (-1)=10) -> (queue out=w181:refnum<queue>, element=w187:cluster{"Mode":T2, T7})  [unwired: 1 in, 2 out]
          n110 = Unbundle(w187) -> ("Mode"=w186:T2, w185:T7)
          n111 = case shown="\"stop\"" w186 {
            tunnel: [_ _ _ TRUE] -> w188
            tunnel: w185 -> [w204 w205 _ _]
            tunnel: [w194 w223 w240 w247] -> w184
            tunnel: w183 -> [_ w223 w240 w247]
            tunnel: w182 -> [_ _ _ _]
            tunnel: w181 -> [w193 w206 w241 w246]
            tunnel: [w193 w207 w241 w246] -> w180
            tunnel: [w190 w213 w237 w245] -> w174
            tunnel: [w191 w215 w238 w244] -> w176
            tunnel: w175 -> [w191 w209 w238 w244]
            tunnel: [w192 w222 w239 w243] -> w179
            tunnel: w178 -> [w192 w222 w239 w243]
            tunnel: w173 -> [w190 w210 w237 w245]
            frame "generateWaves" {
              # "XY Mirrors"
              n112 = Unbundle(w204) -> ("Mode"=w203:enum16{"X", "XY", "XYZ", "XYZT", "XYZC"}, "Piezo Position /um"=w202:dbl, "Exposure/ms"=w199:dbl, "Samples/millisecond"=w201:dbl)  [unwired: 1 out]
              n113 = Reciprocal(x=w199) -> (1/x=w197:dbl)
              n114 = call "XY Galvo With Homography.vi"("Piezo Position (um)"=w203, "Relax (ms)"=w201, "Samples /Millisecond"=w199, "Exposure (ms)"=w202) -> ("Z Mirror Signal"=w198:dbl[], "Scan Mirror Signal"=w200:dbl[])
              n115 = Bundle By Name("Y"=w200, "dt"=w197) -> (w195:waveform(dbl))  [unwired: 1 in]
              n116 = Bundle By Name("Y"=w198, "dt"=w197) -> (w196:waveform(dbl))  [unwired: 1 in]
              n117 = Build Array(w195, w196) -> (w194:waveform(dbl)[])
            }
            frame "runWaves" {
              n118 = Unbundle By Name(w205) -> ("Samples/millisecond"=w226:dbl)  [unwired: 3 out]
              n119 = call-poly <vilib>:"DAQmx Timing.vi"("task/channels in"=w209, "rate"=w226) -> ("task out"=w225:refnum<k21>)  [unwired: 12 in, 1 out]
              n120 = call-poly <vilib>:"DAQmx Timing.vi"("task/channels in"=w210, "rate"=w226) -> ("task out"=w224:refnum<k21>)  [unwired: 12 in, 1 out]
              n121 = call-poly <vilib>:"DAQmx Write.vi"("task/channels in"=w225, "data"=w223) -> ("task out"=w221:refnum<k21>, "error out"=w218:errorcluster)  [unwired: 11 in, 1 out]
              n122 = call-poly <vilib>:"DAQmx Write.vi"("task/channels in"=w224, "data"=w222) -> ("task out"=w220:refnum<k21>, "error out"=w219:errorcluster)  [unwired: 11 in, 1 out]
              n123 = case shown="False" "Scan Continuously" {
                tunnel: w206 -> [w228 w236]
                tunnel: [w229 w235] -> w207
                tunnel: w205 -> [w230 w234]
                frame False {
                  n124 = Bundle("Mode"=ModeEnum."Idle", w230) -> (w231:cluster{"Mode":T2, T7})  [unwired: 1 in]
                  n125 = Enqueue Element(queue=w228, element=w231) -> (queue out=w229:refnum<queue>)  [unwired: 2 in, 2 out]
                }
                frame True {
                  n126 = Bundle("Mode"=ModeEnum."Idle", w234) -> (w233:cluster{"Mode":T2, T7})  [unwired: 1 in]
                  n127 = Enqueue Element(queue=w236, element=w233) -> (queue out=w235:refnum<queue>)  [unwired: 2 in, 2 out]
                }
              }
              n128 = Merge Errors(w218, w219) -> (w217:errorcluster)
              n129 = call <vilib>:"DAQmx Start Task.vi"("task/channels in"=w221, "error in"=w217) -> ("task out"=w216:refnum<k21>, "error out"=w211:errorcluster)  [unwired: 12 in]
              n130 = call <vilib>:"DAQmx Start Task.vi"("task/channels in"=w220, "error in"=w217) -> ("task out"=w214:refnum<k21>, "error out"=w212:errorcluster)  [unwired: 12 in]
              n131 = call <vilib>:"DAQmx Wait Until Done.vi"("task/channels in"=w216, "error in"=w211) -> ("task out"=w215:refnum<k21>)  [unwired: 12 in, 1 out]
              n132 = call <vilib>:"DAQmx Wait Until Done.vi"("task/channels in"=w214, "error in"=w212) -> ("task out"=w213:refnum<k21>)  [unwired: 12 in, 1 out]
            }
            frame "Idle", Default {
            }
            frame "stop" {
            }
          }
        }
        n133 = Merge Errors(w168, w169) -> (w170:errorcluster)
      }
      frame "deinit" {
        n134 = call <vilib>:"DAQmx Stop Task.vi"("task/channels in"=w437) -> ("task out"=w438:refnum<k21>)  [unwired: 13 in, 1 out]
        n135 = call "tm_stopcapture.vi"("error in (no error)"=w449, "Handle in"=w445) -> ("error out"=w452:errorcluster, "Handle out"=w451:u32)  [unwired: 8 in]
        n136 = call <vilib>:"DAQmx Clear Task.vi"("task in"=w438) -> ()  [unwired: 14 in, 1 out]
        n137 = call "tm_unpreparecapture.vi"("error in (no error)"=w452, "Handle in"=w451) -> ("error out"=w453:errorcluster, "Handle out"=w450:u32)  [unwired: 8 in]
        n138 = call "tm_closecamera.vi"("error in (no error)"=w453, "Handle in"=w450) -> ("error out"=w454:errorcluster)  [unwired: 9 in]
        n139 = call "tm_deinitialize.vi"("error in (no error)"=w454) -> ("error out"=w455:errorcluster)  [unwired: 10 in]
        n140 = Release Queue(queue=w443, error in (no error)=w455) -> (error out=w447:errorcluster)  [unwired: 1 in, 2 out]
        n141 = Release Queue(queue=w442, error in (no error)=w455) -> (error out=w446:errorcluster)  [unwired: 1 in, 2 out]
        n142 = Merge Errors(w447, w446) -> (w448:errorcluster)
      }
    }
    n143 = Or(x="stop", y=w24) -> (x .or. y?=w25:bool)
  }
  "error IO" <- w14
  n144 = disable-structure shown="Enabled" {
    frame Disabled {
      # "Parallise decode buffer"
      n145 = call "tm_startcapture_b.vi"() -> ()  [unwired: 10 in, 2 out]
      n146 = call "tm_waitnextframe.vi"() -> ()  [unwired: 8 in, 4 out]
      n147 = call "tm_getframe_a.vi"() -> ()  [unwired: 7 in, 5 out]
    }
    frame Enabled {
    }
  }
